vi "Global - Unit.vi"() -> ()   [LabVIEW 2019]
panel:
  in  "Unit":T1(array[cluster])
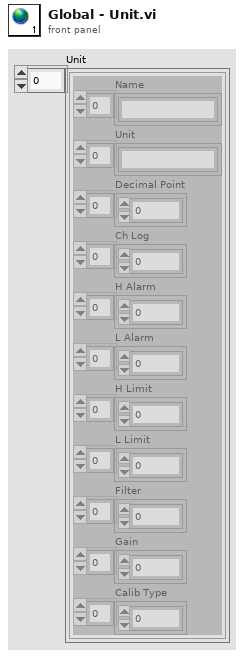
[diagram p1: front panel]
types:
  T1 = cluster{"Name":string[], "Unit":string[], "Decimal Point":u8[], "Ch Log":u8[], "H Alarm":u8[], "L Alarm":u8[], "H Limit":sgl[], "L Limit":sgl[], "Filter":u8[], "Gain":u8[], "Calib Type":u32[]}[]
diagram:
